vi "ReadRegedit.vi"(8 "error in":errorcluster caption="错误输入（无错误）", 10 "名称":string[](array[string]), 11 "subkey":string="SuperJoint\\MyKey") -> (0 "error out":errorcluster caption="错误输出", 2 "值":string[](array[string]))   [LabVIEW 2018]
uses:
  <vilib>/registry/registry.llb/Registry RtKey.ctl
  <vilib>/registry/registry.llb/Read Registry Value Simple STR.vi
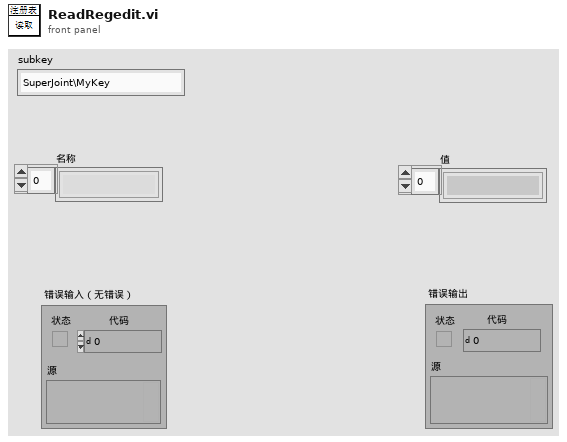
[diagram p1: front panel]
types:
  T1 = typedef "Registry RtKey.ctl" = enum32{"HKEY_CLASSES_ROOT", "HKEY_CURRENT_USER", "HKEY_LOCAL_MACHINE", "HKEY_USERS", "HKEY_PERFORMANCE_DATA", "HKEY_CURRENT_CONFIG", "HKEY_DYN_DATA"}
  T2 = typedef "Registry refnum.ctl" = refnum<k1>
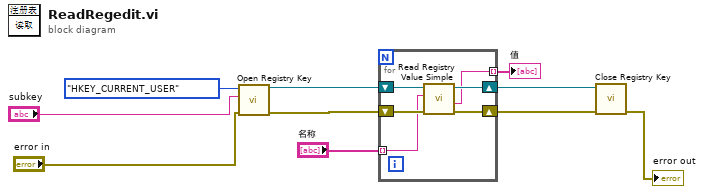
[diagram p0: block diagram]
diagram:
  n1 = call <vilib>:"Open Registry Key.vi"("error in (no error)"="error in", "subkey"="subkey", "root key (HKEY_LOCAL_MACHINE)"=Registry_RtKey."HKEY_CURRENT_USER") -> ("error out"=w7:errorcluster, "refnum out"=w8:T2)  [unwired: 7 in]
  n2 = for {
    shift-right: [w13] -> w5
    shift-left: w8 -> [w16]
    shift-right: [w14] -> w6
    shift-left: w7 -> [w15]
    tunnel: [w12] -> w2 mode=indexing
    tunnel: "名称" -> [w11] mode=indexing
    n3 = call-poly <vilib>:"Read Registry Value Simple.vi"("error in (no error)"=w15, "value"=w11, "refnum"=w16) -> ("error out"=w14:errorcluster, "String/Binary data"=w12:string, "refnum out"=w13:T2)  [unwired: 3 in, 1 out]
  }
  "值" <- w2
  n4 = call <vilib>:"Close Registry Key.vi"("error in (no error)"=w6, "refnum"=w5) -> ("error out"=→"error out":errorcluster)  [unwired: 5 in]
